vi "FileIO-List Parameter Files.vi"(7 "folder":path, 11 "error in (no error)":errorcluster) -> (8 "Parameter file names":string[](array[string]))   [LabVIEW 2020]
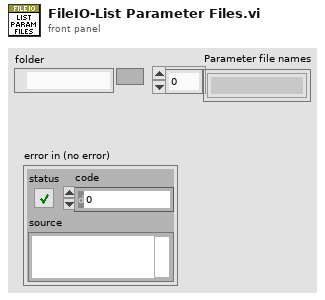
[diagram p1: front panel]
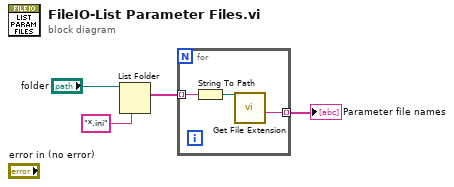
[diagram p0: block diagram]
diagram:
  n1 = List Folder(path="folder", pattern="*.ini") -> (filenames=w2:string[])  [unwired: 2 in, 3 out]
  n2 = for {
    tunnel: w2 -> [w6] mode=indexing
    tunnel: [w5] -> w1 mode=indexing
    n3 = String To Path(string=w6) -> (path=w7:path)
    n4 = call <vilib>:"Get File Extension.vi"("file"=w7) -> ("filename without extension"=w5:string)  [unwired: 6 in, 4 out]
  }
  "Parameter file names" <- w1
